vi "Launch Instruments.vi"(8 "error in":errorcluster, 11 "Manual UI in":refnum<class "Manual UI.lvclass">) -> (0 "error out":errorcluster, 3 "Manual UI out":refnum<class "Manual UI.lvclass">)   [LabVIEW 2023, in "Manual UI.lvlib" / "Manual UI.lvclass"]
uses:
  Project/Manual UI.lvclass
  C:/Users/Public/Documents/Development/builds/Engine/Engine.lvlibp/Project/Engine.lvclass
  Project/Manual UI.lvclass/Manual UI.ctl
  Manual UI Messages/Launch Subordinate and Add Msg/Launch Subordinate and Add Msg.lvclass/Launch Subordinate and Add Msg.ctl
  Manual UI Messages/Update Main State Msg/Update Main State Msg.lvclass/Update Main State Msg.ctl
  Accessors/Read instrPanels.vi
  Accessors/Read Instruments.vi
  builds/Instruments/Instruments.lvlibp/Library/Instruments.lvclass
  C:/Users/Public/Documents/Development/builds/Engine/Actor Framework.lvlibp/1abvi3w/vi.lib/ActorFramework/Actor/Actor.lvclass
  C:/Users/Public/Documents/Development/builds/Engine/Panel Manager.lvlibp/Panel Actor/Panel Actor.lvclass
  builds/Engine/Panel.lvlibp/Panel/Subpanel/Subpanel.lvclass
  C:/Users/Public/Documents/Development/builds/Engine/Panel.lvlibp/Panel/Panel.lvclass
  builds/Engine/Engine.lvlibp/Accessors/Read Report Queue.vi
  builds/Engine/Engine.lvlibp/Accessors/Read Directory.vi
  builds/Engine/Engine.lvlibp/Accessors/Read Events.vi
  builds/Engine/Engine.lvlibp/Accessors/Read Pedigree Val.vi
  builds/Engine/Engine.lvlibp/Accessors/Read Self Q.vi
  builds/Engine/Panel.lvlibp/Panel/Subpanel/Subpanel.vi
  builds/Engine/Engine.lvlibp/Accessors/Write Report Queue.vi
  builds/Instruments/Instruments.lvlibp/Accessors/Write Panel Instruments.vi
  builds/Engine/Actor Framework.lvlibp/1abvi3w/vi.lib/ActorFramework/Actor/Write Actor Label.vi
  builds/Engine/Engine.lvlibp/Accessors/Write Directory.vi
  builds/Engine/Actor Framework.lvlibp/1abvi3w/vi.lib/ActorFramework/Actor/Read Actor Label.vi
  builds/Engine/Engine.lvlibp/Accessors/Write Events.vi
  builds/Engine/Engine.lvlibp/Accessors/Write Pedigree val.vi
  builds/Engine/Actor Framework.lvlibp/1abvi3w/vi.lib/ActorFramework/Message Enqueuer/Enqueue.vi
  builds/Tools/QDMH.lvlibp/QDMH.lvclass
  builds/Engine/Actor Framework.lvlibp/1abvi3w/vi.lib/ActorFramework/Message Enqueuer/Message Enqueuer.lvclass
  Manual UI Messages/Launch Subordinate and Add Msg/Launch Subordinate and Add Msg.lvclass
  Manual UI Messages/Reset Manual Layout Msg/Reset Manual Layout Msg.lvclass
  Manual UI Messages/Update Main State Msg/Update Main State Msg.lvclass
  builds/Engine/Panel.lvlibp
  builds/Engine/Engine.lvlibp/Project/Engine.lvclass
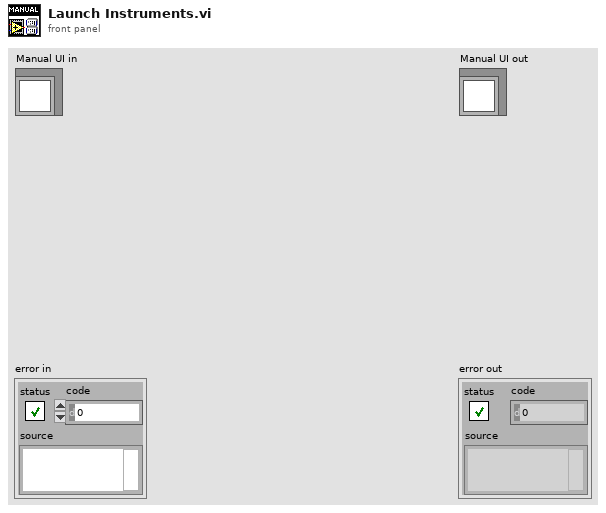
[diagram p1: front panel]
types:
  T1 = typedef "Engine.lvlibp/Engine.lvclass/Engine Events.ctl" = cluster{"System Event":T2, "Manual":T3, "UUT":T4, "Interface Events":T5}
  T2 = typedef "Engine.lvlibp/Engine.lvclass/System Events.ctl" = cluster{"Fault Event":refnum<user-event>, "SystemStatus Event":refnum<user-event>, "Automation":refnum<user-event>}
  T3 = typedef "Engine.lvlibp/Engine.lvclass/Manual Events.ctl" = cluster{"QuickStart Event":refnum<user-event>, "SafeBTE Event":refnum<user-event>, "TogglePower Event":refnum<user-event>, "Change Instrument Event":refnum<user-event>, "Toggle Launch Event":refnum<user-event>, "UUTSupply":refnum<user-event>}
  T4 = typedef "Engine.lvlibp/Engine.lvclass/UUT_Events.ctl" = cluster{"UUT_Name":refnum<user-event>, "Test_Name":refnum<user-event>, "Test_Operator":refnum<user-event>, "Test_Witness":refnum<user-event>, "Pedigree_Event":refnum<user-event>}
  T5 = typedef "Engine.lvlibp/Engine.lvclass/Interface Events.ctl" = cluster{"Interface_Command":refnum<user-event>, "Telemetry_Descriptor":refnum<user-event>, "AsynchTLM_Descriptor":refnum<user-event>}
  T6 = cluster{"Name":string, "Instrument":refnum<class "Instruments.lvclass">, "Panel":i32}[]
  T7 = cluster{"Instrument":refnum<class "Instruments.lvclass">, "Subpanel Out":refnum<class "Subpanel.lvclass">}
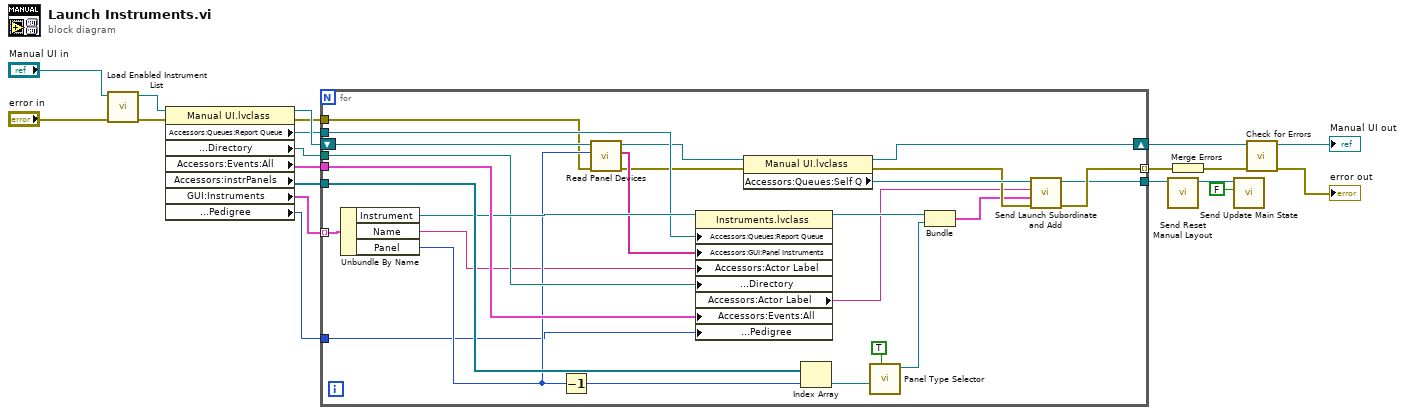
[diagram p0: block diagram]
diagram:
  n1 = call "Load Enabled Instrument List.vi"("error in"="error in", "Manual UI in"="Manual UI in") -> ("error out"=w14:errorcluster, "Manual UI out"=w13:refnum<class "Manual UI.lvclass">)  [unwired: 8 in]
  n2 = property class="Manual UI.lvclass"(reference=w13, error in=w14) -> (reference out=w19:refnum<class "Manual UI.lvclass">, error out=w10:errorcluster, "Accessors:Queues:Report Queue"=w15:refnum<class "QDMH.lvclass">, "Accessors:Application:Information:Directory"=w16:path, "Accessors:Events:All"=w20:T1, "Accessors:instrPanels"=w18:refnum<vi>[], "GUI:Instruments"=w17:T6, "Accessors:Application:Information:Pedigree"=w1:enum16{"STAT", "BB", "PT", "EM", "FT"})
  n3 = for {
    tunnel: w20 -> [w46]
    tunnel: [w26] -> w9 mode=indexing
    tunnel: w18 -> [w43]
    shift-right: [w29] -> w7
    shift-left: w19 -> [w37]
    tunnel: w17 -> [w41] mode=indexing
    tunnel: w16 -> [w39]
    tunnel: w15 -> [w33]
    tunnel: w10 -> [w32]
    tunnel: [w23] -> w8
    tunnel: w1 -> [w21]
    n4 = Unbundle By Name(w41) -> ("Instrument"=w40:refnum<class "Instruments.lvclass">, "Name"=w34:string, "Panel"=w36:i32)
    n5 = Decrement(x=w36) -> (x-1=w22:i32)
    n6 = call "Read Panel Devices.vi"("error in"=w32, "Panel Index"=w36, "Manual UI in"=w37) -> ("error out"=w30:errorcluster, "Panel Devices"=w35:string[], "Manual UI out"=w31:refnum<class "Manual UI.lvclass">)  [unwired: 6 in]
    n7 = property class="Instruments.lvclass"(reference=w40, "Accessors:Queues:Report Queue"=w33, "Accessors:GUI:Panel Instruments"=w35, "Accessors:Actor Label"=w34, "Accessors:Application:Information:Directory"=w39, "Accessors:Events:All"=w46, "Accessors:Application:Information:Pedigree"=w21) -> (reference out=w45:refnum<class "Instruments.lvclass">, "Accessors:Actor Label"=w24:string)  [unwired: 1 in, 1 out]
    n8 = property class="Manual UI.lvclass"(reference=w31, error in=w30) -> (reference out=w29:refnum<class "Manual UI.lvclass">, error out=w27:errorcluster, "Accessors:Queues:Self Q"=w28:refnum<class "Message Enqueuer.lvclass">)
    n9 = Index Array(array=w43, index=w22) -> (element=w42:refnum<vi>)
    n10 = call-poly "Panel Type Selector.vi"("Autoshow? (T)"=TRUE, "Sub Panel"=w42) -> ("Subpanel Out"=w44:refnum<class "Subpanel.lvclass">)  [unwired: 8 in, 1 out]
    n11 = Bundle("Instrument"=w45, "Subpanel Out"=w44) -> (w25:T7)  [unwired: 1 in]
    n12 = call "Send Launch Subordinate and Add.vi"("error in (no error)"=w27, "Panel Definiton"=w25, "Identifier"=w24, "Message Enqueuer"=w28) -> ("error out"=w26:errorcluster, "Message Enqueuer out"=w23:refnum<class "Message Enqueuer.lvclass">)  [unwired: 6 in]
  }
  n13 = call "Send Reset Manual Layout.vi"("Message Enqueuer"=w8) -> ("Message Enqueuer out"=w3:refnum<class "Message Enqueuer.lvclass">)  [unwired: 9 in, 1 out]
  n14 = Merge Errors(w9) -> (w6:errorcluster)
  n15 = call "Send Update Main State.vi"("Loading"=FALSE, "Message Enqueuer"=w3) -> ()  [unwired: 8 in, 2 out]
  n16 = call "Check for Errors.vi"("error in"=w6, "Engine in"=w7) -> ("error out"=→"error out":errorcluster, "Engine out"=→"Manual UI out":refnum<class "Manual UI.lvclass">)  [unwired: 8 in]
